vi "Update Operating Mode.vi"(10 "UTP IO Session in":T1, 11 "Sequence Context In":refnum<k7>) -> ()   [LabVIEW 2023]
uses:
  <vilib>/Noffz/UTP IO/UTP IO Library/Typedefs/Session Handle.ctl
  <vilib>/Noffz/UTP IO/UTP IO Library/UTP IO Pool Session.lvclass
  <vilib>/Noffz/UTP IO/UTP IO Library/methods/poly/plc/Read PLC Variable (I16).vi
  <vilib>/addons/TestStand/_TSUtility.llb/TestStand - Set Property Value (Number {Signed 16-bit Integer}).vi
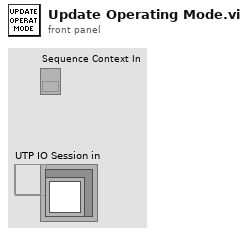
[diagram p1: front panel]
types:
  T1 = typedef "UTP IO Library.lvlib/UTP IO Pool Session.lvclass/Session Handle.ctl" = refnum<data-value>
  T2 = typedef "TestStand - Status Monitor.ctl" = cluster{"Sequence Context":refnum<k7>, "Execution":refnum<k7>, "Termination Monitor":refnum<k7>}
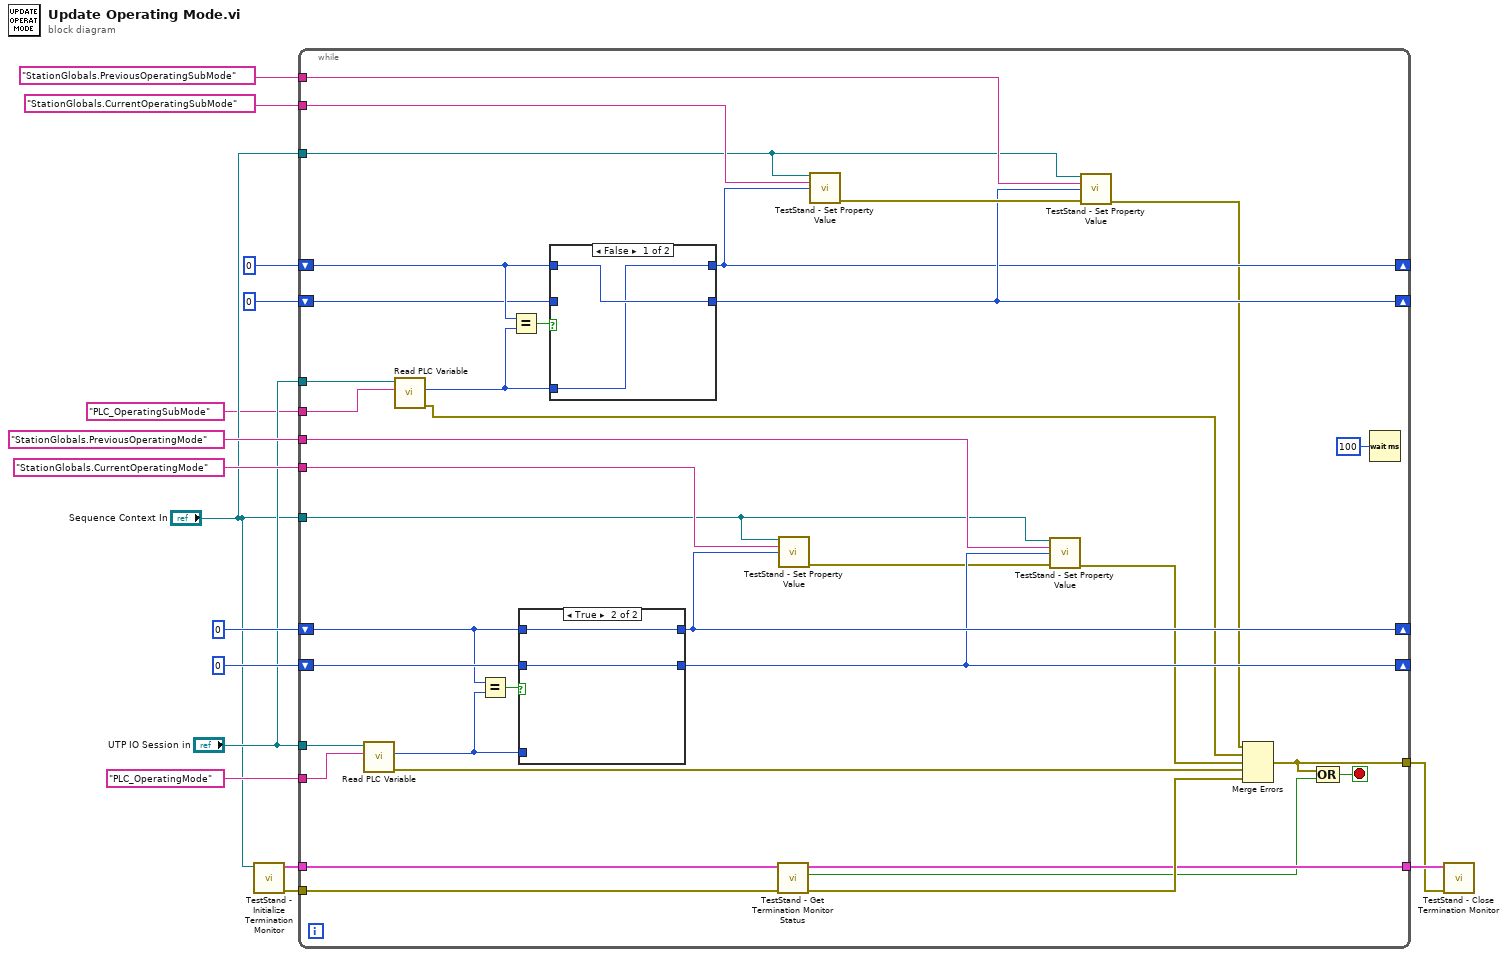
[diagram p0: block diagram]
diagram:
  n1 = call <vilib>:"TestStand - Initialize Termination Monitor.vi"("Sequence Context In"="Sequence Context In") -> ("error out"=w13:errorcluster, "Status Monitor Out"=w12:T2)  [unwired: 9 in]
  n2 = while {
    tunnel: "UTP IO Session in" -> [w52]
    tunnel: "PLC_OperatingMode" ("variable name") -> [w51]
    shift-right: [w45] -> _
    shift-left: i16 0 ("value") -> [w47]
    shift-right: [w44] -> _
    shift-left: i16 0 ("value") -> [w48]
    tunnel: "Sequence Context In" -> [w21]
    tunnel: w13 -> [w42]
    tunnel: w12 -> [w41]
    tunnel: [w37] -> w11
    tunnel: [w35] -> w10
    tunnel: "StationGlobals.CurrentOperatingMode" ("Lookup String") -> [w33]
    tunnel: "StationGlobals.PreviousOperatingMode" ("Lookup String") -> [w32]
    tunnel: "UTP IO Session in" -> [w22]
    shift-right: [w27] -> _
    shift-left: i16 0 ("value") -> [w26]
    shift-right: [w28] -> _
    shift-left: i16 0 ("value") -> [w25]
    tunnel: "StationGlobals.CurrentOperatingSubMode" ("Lookup String") -> [w30]
    tunnel: "StationGlobals.PreviousOperatingSubMode" ("Lookup String") -> [w31]
    tunnel: "Sequence Context In" -> [w20]
    tunnel: "PLC_OperatingSubMode" ("variable name") -> [w19]
    stop <- w36 stop-if-true
    n3 = call-poly <vilib>:"Read PLC Variable.vi"("variable name"=w51, "UTP IO Session in"=w52) -> ("error out"=w39:errorcluster, "value"=w49:i16)  [unwired: 7 in, 1 out]
    n4 = call-poly <vilib>:"Read PLC Variable.vi"("variable name"=w19, "UTP IO Session in"=w22) -> ("error out"=w17:errorcluster, "value"=w24:i16)  [unwired: 7 in, 1 out]
    n5 = Equal?(x=w47, y=w49) -> (x = y?=w50:bool)
    n6 = Equal?(x=w26, y=w24) -> (x = y?=w23:bool)
    n7 = case shown="True" w50 {
      tunnel: w49 -> [w57 _]
      tunnel: [w57 w59] -> w45
      tunnel: [w58 w60] -> w44
      tunnel: w48 -> [_ w60]
      tunnel: w47 -> [w58 w59]
      frame False {
      }
      frame True {
      }
    }
    n8 = case shown="False" w23 {
      tunnel: w24 -> [w53 _]
      tunnel: [w53 w55] -> w27
      tunnel: [w54 w56] -> w28
      tunnel: w25 -> [_ w56]
      tunnel: w26 -> [w54 w55]
      frame False {
      }
      frame True {
      }
    }
    n9 = call <vilib>:"TestStand - Get Termination Monitor Status.vi"("error in (no error)"=w42, "Status Monitor In"=w41) -> ("error out"=w38:errorcluster, "Terminating or Aborting"=w34:bool, "Status Monitor Out"=w37:T2)  [unwired: 7 in]
    n10 = call-poly <vilib>:"TestStand - Set Property Value.vi"("Sequence Context In"=w21, "Lookup String"=w33, "New Value"=w45) -> ("error out"=w43:errorcluster)  [unwired: 11 in, 1 out]
    n11 = call-poly <vilib>:"TestStand - Set Property Value.vi"("Sequence Context In"=w20, "Lookup String"=w30, "New Value"=w27) -> ("error out"=w29:errorcluster)  [unwired: 11 in, 1 out]
    n12 = call-poly <vilib>:"TestStand - Set Property Value.vi"("Sequence Context In"=w21, "Lookup String"=w32, "New Value"=w44, "error in (no error)"=w43) -> ("error out"=w40:errorcluster)  [unwired: 10 in, 1 out]
    n13 = call-poly <vilib>:"TestStand - Set Property Value.vi"("Sequence Context In"=w20, "Lookup String"=w31, "New Value"=w28, "error in (no error)"=w29) -> ("error out"=w18:errorcluster)  [unwired: 10 in, 1 out]
    n14 = Merge Errors(w18, w17, w40, w39, w38) -> (w35:errorcluster)
    n15 = Compound Arithmetic op=OR(w35, w34) -> (w36:bool)
    n16 = Wait (ms)(milliseconds to wait=u32 100) -> ()  [unwired: 1 out]
  }
  n17 = call <vilib>:"TestStand - Close Termination Monitor.vi"("error in (no error)"=w10, "Status Monitor In"=w11) -> ()  [unwired: 9 in, 1 out]
